vi "Checker(sub).vi"(7 "Path of File":path=path "C:/Users/KimYG/Desktop/test4.abf") -> (3 "배열 2":i32[](array[numeric]))   [LabVIEW 2017]
uses:
  Minhee Retriever/Polarity.ctl
  Data type_new.ctl
  Minhee analysis parameter setting.ctl
  <vilib>/Analysis/3filter.llb/Savitzky-Golay Filter (DBL).vi
  <vilib>/addons/Wavelet Analysis/application.llb/WA Multiscale Peak Detection (Array).vi
  <vilib>/Analysis/NI_AALBase.lvlib
  <vilib>/addons/_Advanced Signal Processing/NI_AdvSigProcWA.lvlib
panel:
  in  "배열":T1[](array[typedef]) {"Screening threshold (amplitude)" format="%#_13g"; "Event Detection Parameter"."Threshold" format="%#_13g"}
  in  "Data type":T2 items=["AXON", "HEKA"]
  in  "Polarity":T3 items=["Inward", "Outward"]
  in  "Sweep length":dbl=51662.0
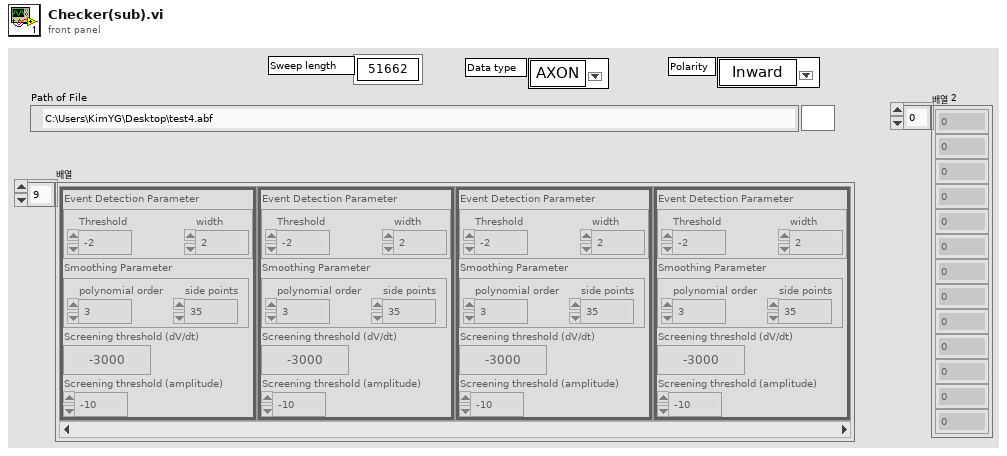
[diagram p1: front panel]
types:
  T1 = typedef "Minhee analysis parameter setting.ctl" = cluster{"Event Detection Parameter":cluster{"Threshold":dbl, "width ":i32}, "Smoothing Parameter":cluster{"polynomial order":i32, "side points":i32}, "Screening threshold (dV/dt)":dbl, "Screening threshold (amplitude)":dbl}
  T2 = typedef "Data type_new.ctl" = u16
  T3 = typedef "Polarity.ctl" = u16
  T4 = cluster{"detrend? (F)":bool, "threshold frequency":dbl}
  T5 = cluster{"File Path":path, "Cell ID":string, "File Name":string, "Total Length":i32, "Trial Length (ms)":dbl, "Sweep Number":dbl, "Sampling rate":dbl}
  T6 = cluster{"polynomial order":i32, "side points":i32}
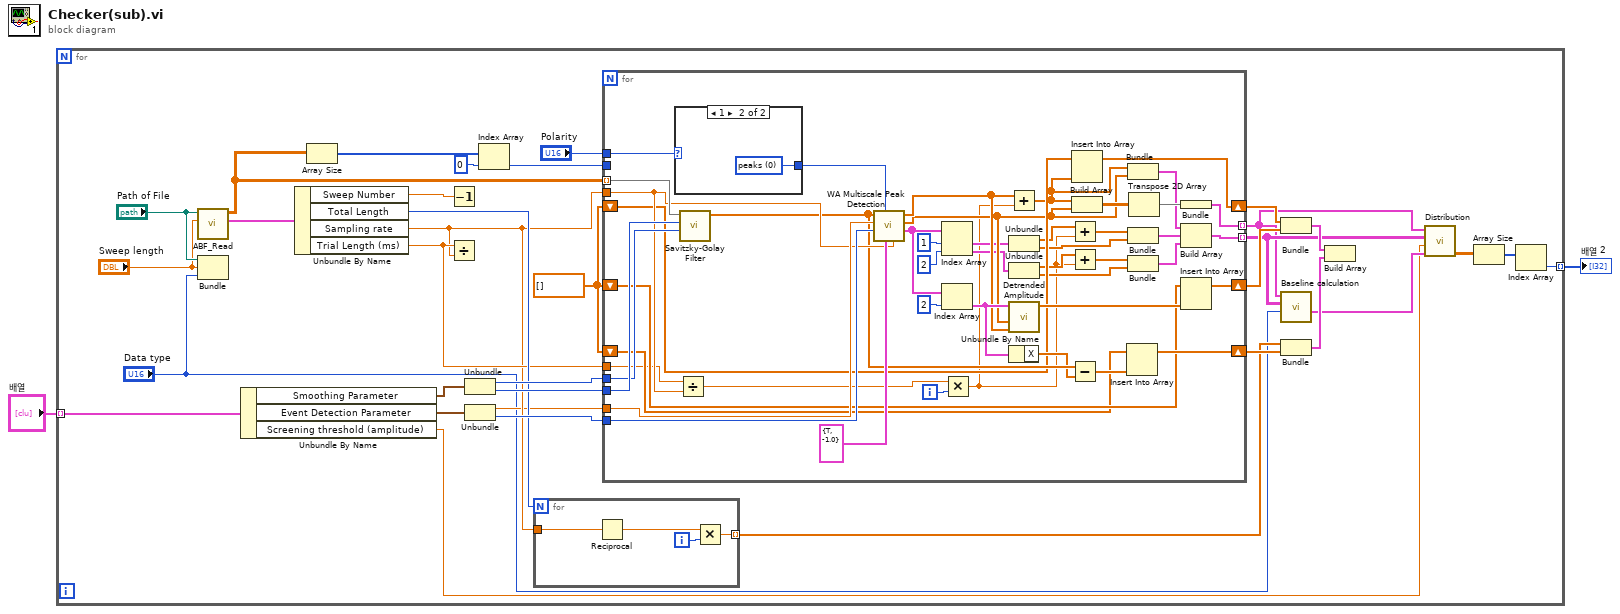
[diagram p0: block diagram]
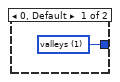
[diagram p2: hidden frame]
diagram:
  n1 = for {
    tunnel: "배열" -> [w13] mode=indexing
    tunnel: [w3] -> w1 mode=indexing
    w36 = dbl[] []
    n2 = call "ABF_Read.vi"("Trial Length (ms)"="Sweep length", "Path of ABF file"="Path of File") -> ("File Paramters"=w10:T5, "Whole Trace"=w22:dbl[][])  [unwired: 2 in, 2 out]
    n3 = Bundle("Path of File"="Path of File", "Sweep length"="Sweep length", "Data type"="Data type") -> ()  [unwired: 1 in, 1 out]
    n4 = Unbundle By Name(w13) -> ("Smoothing Parameter"=w28:T6, "Event Detection Parameter"=w30:cluster{"Threshold":dbl, "width ":i32}, "Screening threshold (amplitude)"=w6:dbl)
    n5 = Unbundle By Name(w10) -> ("Sweep Number"=w21:dbl, "Total Length"=w20:i32, "Sampling rate"=w17:dbl, "Trial Length (ms)"=w18:dbl)
    n6 = Array Size(array=w22) -> (size(s)=w25:i32[])
    n7 = Decrement(x=w21) -> ()  [unwired: 1 out]
    n8 = Divide(x=w18, y=w17) -> ()  [unwired: 1 out]
    n9 = Unbundle(w28) -> ("polynomial order"=w27:i32, "side points"=w26:i32)
    n10 = Unbundle(w30) -> ("Threshold"=w12:dbl, "width"=w29:i32)
    n11 = Index Array(array=w25, index=0 ("인덱스")) -> (element=w23:i32)
    n12 = for {
      N: w20 -> [_]
      tunnel: w17 -> [w40]
      tunnel: [w37] -> w19 mode=indexing
      i -> [w38]
      n13 = Reciprocal(x=w40) -> (1/x=w39:dbl)
      n14 = Multiply(x=w39, y=w38) -> (x*y=w37:dbl)
    }
    n15 = for {
      tunnel: w22 -> [w86] mode=indexing
      tunnel: w17 -> [w78]
      tunnel: w26 -> [w83]
      tunnel: w27 -> [w82]
      tunnel: [w44] -> w9 mode=indexing
      tunnel: w12 -> [w81]
      tunnel: w29 -> [w80]
      shift-right: [w75] -> w35
      shift-left: w36 -> [w67]
      shift-right: [w79] -> w34
      shift-left: w36 -> [w68]
      shift-right: [w62] -> w33
      shift-left: w36 -> [w69]
      tunnel: w18 -> [w59]
      tunnel: [w63] -> w8 mode=indexing
      tunnel: w23 -> [_]
      tunnel: "Polarity" -> [w41]
      i -> [w42]
      n16 = case shown="1" w41 {
        tunnel: [w87 w88] -> w85
        frame 0, Default {
          w87 = u16 1 items=["peaks", "valleys"] ("peaks/valleys")
        }
        frame 1 {
          w88 = u16 0 items=["peaks", "valleys"] ("peaks/valleys")
        }
      }
      n17 = Divide(x=w59, y=w78) -> (x/y=w77:dbl)
      n18 = call-poly <vilib>:"Savitzky-Golay Filter.vi"("polynomial order"=w82, "side points"=w83, "X"=w86) -> ("Filtered X"=w74:dbl[])  [unwired: 7 in, 1 out]
      n19 = call-poly <vilib>:"WA Multiscale Peak Detection.vi"("sampling rate"=w78, "detrend settings"=T4 {"detrend? (F)"=TRUE, "threshold frequency"=-1.0}, "peaks/valleys"=w85, "width"=w80, "threshold"=w81, "signal"=w74) -> ("peak plot"=w58:cluster{"Ramp Pattern":dbl[], "X":dbl[]}[], "amplitude"=w60:dbl[], "location"=w66:dbl[])  [unwired: 1 in, 2 out]
      n20 = Index Array(array=w58, index #1=1 ("인덱스"), index #2=2 ("인덱스")) -> (element #1=w56:cluster{"Ramp Pattern":dbl[], "X":dbl[]}, element #2=w51:cluster{"Ramp Pattern":dbl[], "X":dbl[]})
      n21 = Index Array(array=w58, index=2 ("인덱스")) -> (element=w71:cluster{"Ramp Pattern":dbl[], "X":dbl[]})
      n22 = Multiply(x=w77, y=w42) -> (x*y=w43:dbl)
      n23 = Add(x=w66, y=w43) -> (x+y=w61:dbl[])
      n24 = Unbundle(w56) -> ("Ramp Pattern"=w55:dbl[], "X"=w53:dbl[])
      n25 = Unbundle(w51) -> ("Ramp Pattern"=w50:dbl[], "X"=w48:dbl[])
      n26 = call "Detrended Amplitude.vi"("location"=w66, "Amplitude"=w60, "Trend"=w71) -> ("detrended amplitude"=w70:dbl[])  [unwired: 4 in]
      n27 = Unbundle By Name(w71) -> ("X"=w72:dbl[])
      n28 = Add(x=w55, y=w43) -> (x+y=w54:dbl[])
      n29 = Add(x=w50, y=w43) -> (x+y=w49:dbl[])
      n30 = Subtract(x=w74, y=w72) -> (x-y=w73:dbl[])
      n31 = Insert Into Array(array=w69, new element=w61) -> (w62:dbl[])  [unwired: 1 in]
      n32 = Build Array(w61, w60) -> (w65:dbl[][])
      n33 = Insert Into Array(array=w67, new element=w73) -> (w75:dbl[])  [unwired: 1 in]
      n34 = Bundle(w61, "amplitude"=w60) -> (w45:cluster{dbl[], "amplitude":dbl[]})  [unwired: 1 in]
      n35 = Bundle(w54, "X"=w53) -> (w46:cluster{dbl[], "X":dbl[]})  [unwired: 1 in]
      n36 = Bundle(w49, "X"=w48) -> (w47:cluster{dbl[], "X":dbl[]})  [unwired: 1 in]
      n37 = Transpose 2D Array(2D array=w65) -> (transposed array=w64:dbl[][])
      n38 = Bundle(w64) -> (w63:cluster{dbl[][]})  [unwired: 1 in]
      n39 = Build Array(w45, w46, w47) -> (w44:cluster{dbl[], "X":dbl[]}[])
      n40 = Insert Into Array(array=w68, new element=w70) -> (w79:dbl[])  [unwired: 1 in]
    }
    n41 = Bundle(w33, w34) -> (w31:cluster{dbl[], dbl[]})  [unwired: 1 in]
    n42 = call "Baseline calculation.vi"("Data type"="Data type", "Sweep trace (2D) In"=w9, "Detected Event (1D) In"=w8) -> ("New Baseline info"=w7:cluster{dbl[][]}[])  [unwired: 3 in, 1 out]
    n43 = Bundle(w19, w35) -> (w32:cluster{dbl[], dbl[]})  [unwired: 1 in]
    n44 = Build Array(w31, w32) -> ()  [unwired: 1 out]
    n45 = call "Distribution.vi"("Detected Event (1D)"=w8, "Sweep trace (2D) In"=w9, "Threshold"=w6, "Baseline info new"=w7) -> ("Event final"=w5:dbl[][])  [unwired: 4 out]
    n46 = Array Size(array=w5) -> (size(s)=w4:i32[])
    n47 = Index Array(array=w4) -> (element=w3:i32)  [unwired: 1 in]
  }
  "배열 2" <- w1
